vi "Disdrometer_ReadConfigFile.vi"(8 "ErrorIn":errorcluster, 11 "User":T1={"Port"="Port2", "SNR Threshold"=0.0, "FileFolder"=path "C:/ConnexData"}) -> (0 "ErrorOut":errorcluster, 2 "dup path":path, 3 "User":T1={"Port"="Port2", "SNR Threshold"=0.0, "FileFolder"=path "C:/ConnexData"})   [LabVIEW 2018]
doc: "Attempt to read the configuration (INI) file specified in ClusterIn.Paths.CfgFile. If the file exists, the INI file is read and elements are filled in to the cluster. If it does not exist, a new INI file is created using default values.\n\nAdd elements to this VI for each cluster element that you wish to reload.\n\nCopyright © 2019 Epimedia, Inc. All Rights Reserved.\n\nThe Epimedia Application Library is Copyright © 2009-2017 Epimedia, Inc. \nAll Rights Reserved. Used under license."
uses:
  Disdrometer_UserDefined_clust.ctl
  <vilib>/Utility/sysdir.llb/System Directory Type.ctl
  <vilib>/Utility/xml.llb/Read From XML File(string).vi
panel:
  # "Copyright © 2019 Epimedia, Inc. All Rights Reserved.\n\nThe Epimedia Application Library is Copyright © 2009-2017 Epimedia, Inc. \nAll Rights Reserved. Used under license."
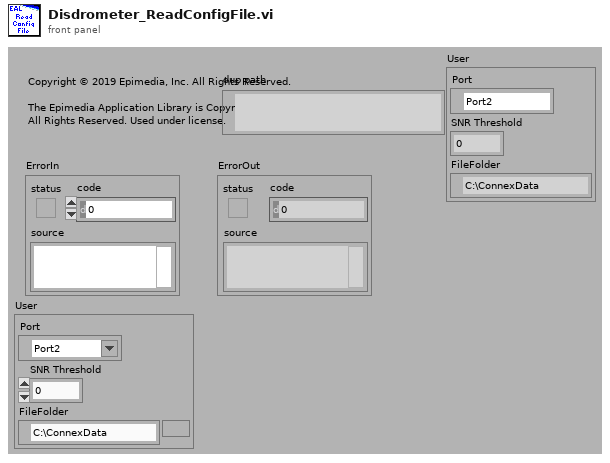
[diagram p1: front panel]
types:
  T1 = typedef "Disdrometer_UserDefined_clust.ctl" = cluster{"Port":refnum<visa-resource-name>, "SNR Threshold":dbl, "FileFolder":path}
  T2 = typedef "System Directory Type.ctl" = i32
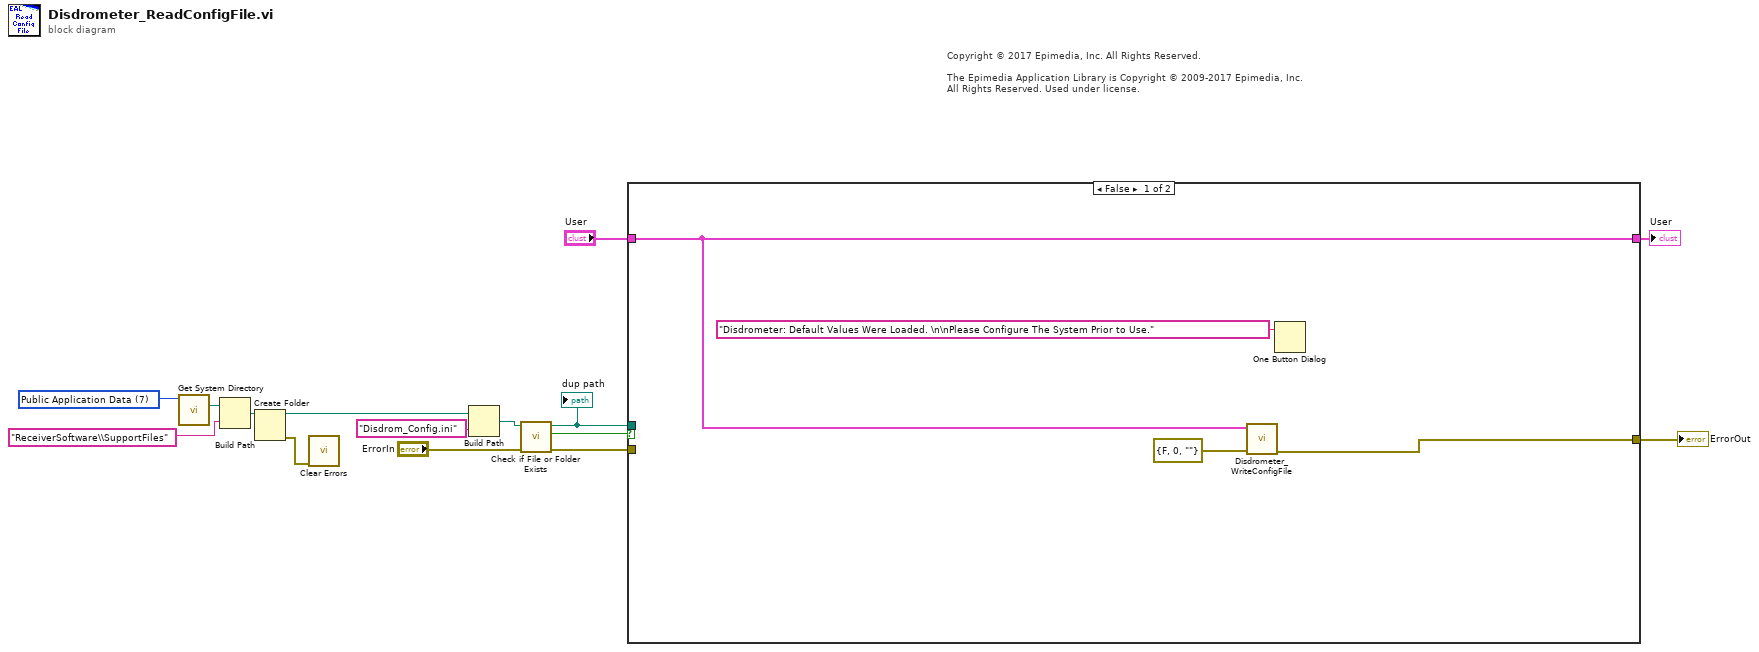
[diagram p0: block diagram]
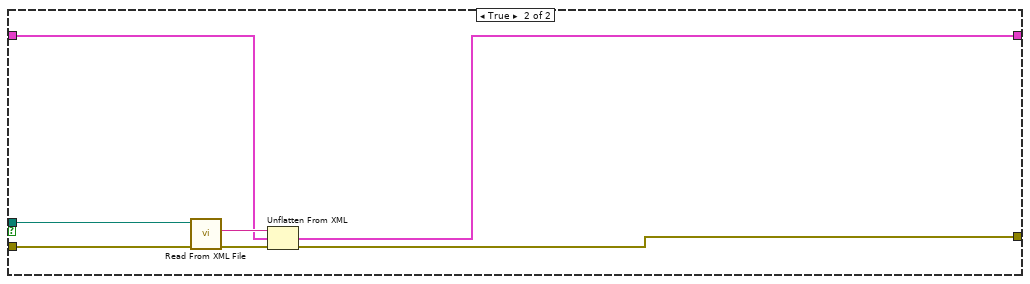
[diagram p2: hidden frame]
diagram:
  w6 = T2 7 items=["User Home"=0, "User Desktop"=1, "User Documents"=2, "User Application Data"=3, "User Preferences"=4, "User Temporary"=5, "Public Documents"=6, "Public Application Data"=7, "Public Preferences"=8, "Public Cache"=13, "System Core Libraries"=9, "System Installed Libraries"=10, "Application Files"=11, "Boot Volume Root"=12] ("system directory type")
  # "Copyright © 2017 Epimedia, Inc. All Rights Reserved.\n\nThe Epimedia Application Library is Copyright © 2009-2017 Epimedia, Inc. \nAll Rights Reserved. Used under license."
  n1 = call <vilib>:"Get System Directory.vi"("system directory type"=w6) -> ("system directory"=w8:path)  [unwired: 10 in]
  n2 = Build Path(base path=w8, name or relative path="ReceiverSoftware\\SupportFiles") -> (appended path=w9:path)
  n3 = Create Folder(path (use dialog)=w9) -> (created path=w5:path, error out=w1:errorcluster)  [unwired: 2 in, 1 out]
  n4 = call <vilib>:"Clear Errors.vi"("error in (no error)"=w1) -> ()  [unwired: 5 in, 2 out]
  n5 = Build Path(base path=w5, name or relative path="Disdrom_Config.ini") -> (appended path=w3:path)
  n6 = call <vilib>:"Check if File or Folder Exists.vi"("error in (no error)"="ErrorIn", "path"=w3) -> ("error out"=w11:errorcluster, "file or folder exists?"=w12:bool, "dup path"=w13:path)  [unwired: 7 out]
  "dup path" <- w13
  n7 = case shown="False" w12 {
    tunnel: [w18 w23] -> w15
    tunnel: [w16 w26] -> w2
    tunnel: w13 -> [_ w25]
    tunnel: "User" -> [w16 w20]
    tunnel: w11 -> [_ w24]
    frame False {
      n8 = call "Disdrometer_WriteConfigFile.vi"("ErrorIn"=errorcluster {"status"=FALSE, "code"=0, "source"=""}, "User"=w16) -> ("ErrorOut"=w18:errorcluster)  [unwired: 9 in]
      n9 = One Button Dialog(message="Disdrometer: Default Values Were Loaded. \n\nPlease Configure The System Prior to Use.") -> ()  [unwired: 2 out]
    }
    frame True {
      n10 = call-poly <vilib>:"Read From XML File.vi"("error in (no error)"=w24, "XML File Path"=w25) -> ("error out"=w22:errorcluster, "XML Elements"=w21:string)  [unwired: 7 in, 1 out]
      n11 = Unflatten From XML(xml string=w21, type=w20, error in (no error)=w22) -> (value=w26:T1, error out=w23:errorcluster)
    }
  }
  "ErrorOut" <- w15
  "User" <- w2
